vi "TDMS_ReadEveryGap.vi"(7 "游标设定":T1={"初始Offset"=0, "每隔多少点读一次"=100000, "每次读的点数"=1}, 8 "错误输入":errorcluster, 9 "通道名":string[](array[string])=["Sinc", "Sin"], 10 "组名称输入":string="Sig Group", 11 "tdms文件":refnum<k34>) -> (0 "错误输出":errorcluster, 1 "二维数组":dbl[][](graph), 2 "队列Ref数组":refnum<queue>[](array[refnum]), 3 "tdms file out":refnum<k34>)   [LabVIEW 2011]
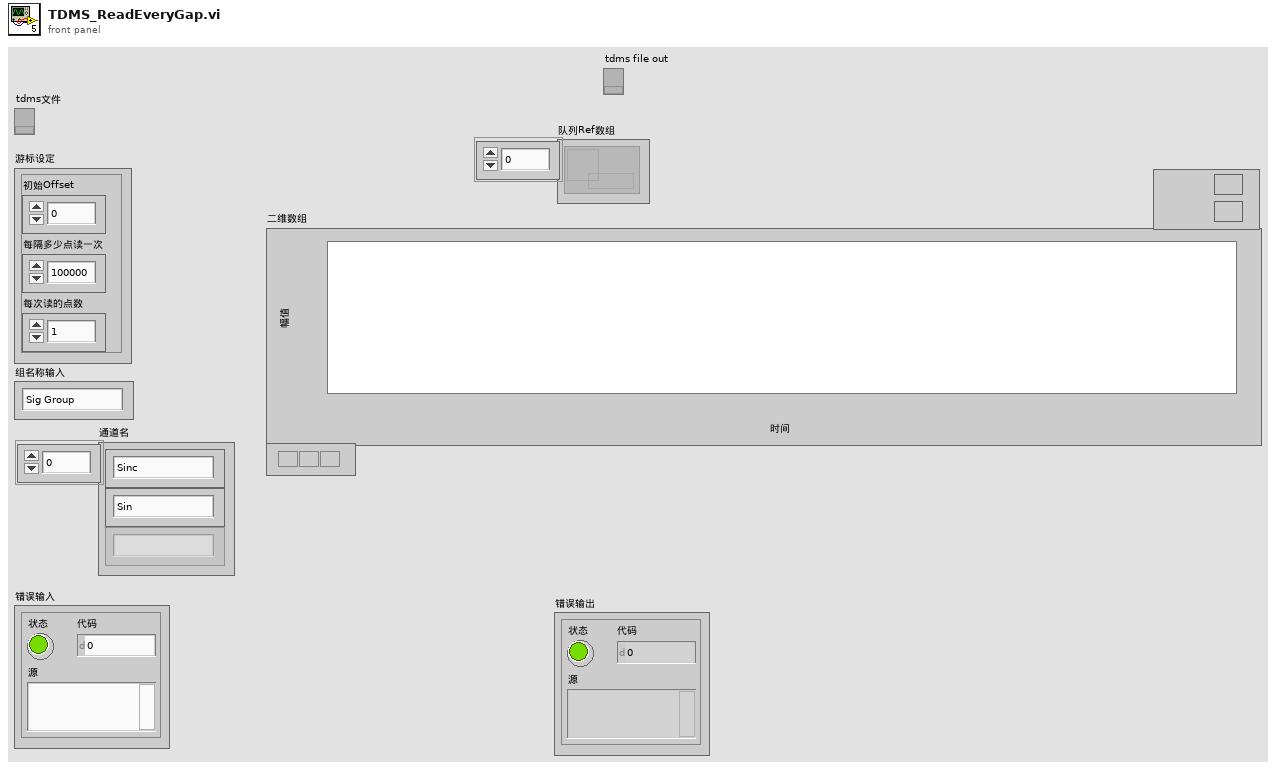
[diagram p1: front panel]
types:
  T1 = cluster{"初始Offset":u64, "每隔多少点读一次":u64, "每次读的点数":u64}
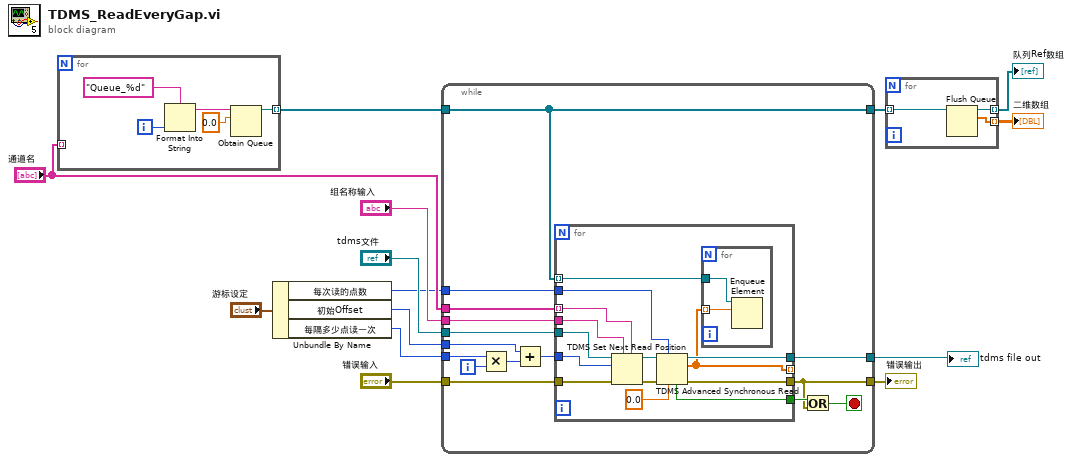
[diagram p0: block diagram]
diagram:
  n1 = for {
    tunnel: "通道名" -> [_] mode=indexing
    tunnel: [w19] -> w13 mode=indexing
    i -> [w18]
    n2 = Format Into String(format string="Queue_%d" ("格式字符串"), w18) -> (resulting string=w17:string)  [unwired: 2 in, 1 out]
    n3 = Obtain Queue(name (unnamed)=w17, element data type=0.0) -> (queue out=w19:refnum<queue>)  [unwired: 3 in, 2 out]
  }
  n4 = Unbundle By Name("游标设定") -> ("每次读的点数"=w4:u64, "初始Offset"=w2:u64, "每隔多少点读一次"=w3:u64)
  n5 = while {
    tunnel: "组名称输入" -> [w22]
    tunnel: "通道名" -> [w26]
    tunnel: "tdms文件" -> [w25]
    tunnel: w3 -> [w30]
    tunnel: w2 -> [w28]
    tunnel: w4 -> [w32]
    tunnel: [w31] -> w1
    tunnel: "错误输入" -> [w23]
    tunnel: w13 -> [w21]
    tunnel: [w21] -> w12
    tunnel: [w20] -> w6
    i -> [w29]
    stop <- w34 stop-if-true
    n6 = Multiply(x=w30, y=w29) -> (x*y=w27:u64)
    n7 = Add(x=w28, y=w27) -> (x+y=w24:u64)
    n8 = for {
      tunnel: [w48] -> w33
      tunnel: w32 -> [w47]
      tunnel: [w46] -> w20
      tunnel: [w45] -> w31
      tunnel: w26 -> [w38] mode=indexing
      tunnel: w25 -> [w43]
      tunnel: w24 -> [w42]
      tunnel: w23 -> [w41]
      tunnel: w22 -> [w37]
      tunnel: [w35] -> _ mode=indexing
      tunnel: w21 -> [w36] mode=indexing
      n9 = TDMS Set Next Read Position(5:w38, 7:w37, 8:w41, 10:w42, 11:w43) -> (0:w40:errorcluster, 3:w39:refnum<k34>)  [unwired: 1 in]
      n10 = TDMS Advanced Synchronous Read(6:0.0, 7:w47, 8:w40, 11:w39) -> (0:w46:errorcluster, 2:w35:dbl[], 3:w45:refnum<k34>, 4:w48:bool)
      n11 = for {
        tunnel: w36 -> [w50]
        tunnel: w35 -> [w49] mode=indexing
        n12 = Enqueue Element(queue=w50, element=w49) -> ()  [unwired: 2 in, 3 out]
      }
    }
    n13 = Or(x=w33, y=w20) -> (x .or. y?=w34:bool)
  }
  "错误输出" <- w6
  "tdms file out" <- w1
  n14 = for {
    tunnel: w12 -> [w53] mode=indexing
    tunnel: [w52] -> w11 mode=indexing
    tunnel: [w51] -> w7 mode=indexing
    n15 = Flush Queue(queue=w53) -> (queue out=w51:refnum<queue>, remaining elements=w52:dbl[])  [unwired: 1 in, 1 out]
  }
  "二维数组" <- w11
  "队列Ref数组" <- w7
